vi "WriteString.vi"(8 "error in (no error)":errorcluster, 10 "Data":string, 11 "UUTIndex":string) -> (0 "error out":errorcluster)   [LabVIEW 2018]
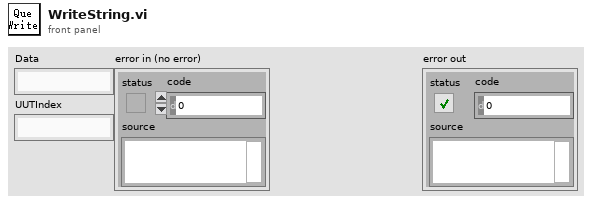
[diagram p1: front panel]
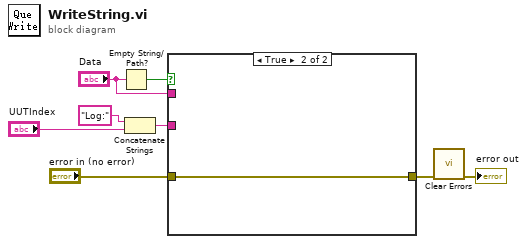
[diagram p0: block diagram]
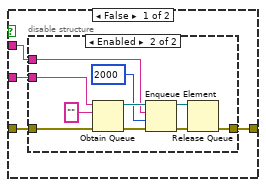
[diagram p2: hidden frame]
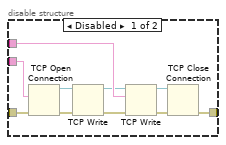
[diagram p3: hidden frame]
diagram:
  n1 = Empty String/Path?(string/path="Data") -> (empty?=w1:bool)
  n2 = Concatenate Strings("Log:" ("string"), "UUTIndex") -> (w3:string)
  n3 = case shown="True" w1 {
    tunnel: [w12 w34] -> w8
    tunnel: "error in (no error)" -> [w11 w34]
    tunnel: w3 -> [w10 _]
    tunnel: "Data" -> [w9 _]
    frame False {
      n4 = disable-structure shown="Enabled" {
        disable-tunnel: [w21 w28] -> w12
        disable-tunnel: w9 -> [w19 w29]
        disable-tunnel: w10 -> [w14 w33]
        disable-tunnel: w11 -> [w13 w32]
        frame Disabled {
          n5 = TCP Open Connection(remote port or service name=w14, error in (no error)=w13) -> (connection ID=w16:refnum<k5>, error out=w15:errorcluster)  [unwired: 3 in]
          n6 = TCP Write(connection ID=w16, error in (no error)=w15) -> (data in=w20:string, connection ID out=w17:refnum<k5>, error out=w18:errorcluster)  [unwired: 2 out]
          n7 = TCP Write(connection ID=w17, data in=w19, error in (no error)=w18) -> (connection ID out=w23:refnum<k5>, error out=w22:errorcluster)  [unwired: 2 out]
          n8 = TCP Close Connection(connection ID=w23, error in (no error)=w22) -> (error out=w21:errorcluster)  [unwired: 2 out]
        }
        frame Enabled {
          n9 = Obtain Queue(name (unnamed)=w33, element data type="", error in (no error)=w32) -> (queue out=w31:refnum<queue>, error out=w30:errorcluster)  [unwired: 2 in, 1 out]
          n10 = Enqueue Element(queue=w31, element=w29, timeout in ms (-1)=2000, error in (no error)=w30) -> (queue out=w27:refnum<queue>, error out=w26:errorcluster)  [unwired: 1 out]
          n11 = Release Queue(queue=w27, error in (no error)=w26) -> (error out=w28:errorcluster)  [unwired: 1 in, 2 out]
        }
      }
    }
    frame True {
    }
  }
  n12 = call <vilib>:"Clear Errors.vi"("error in (no error)"=w8) -> ("error out"=→"error out":errorcluster)  [unwired: 5 in, 1 out]
